vi "Update Graphs.vi"(8 "error in (no error)":errorcluster, 10 "image":variant[][](array[variant]), 11 "Detail Graph in":refnum<class "Detail Graph.lvclass">) -> (0 "error out":errorcluster, 1 "Cursor.Cursor Position":T1, 3 "Detail Graph out":refnum<class "Detail Graph.lvclass">)   [LabVIEW 2023, in "Detail Graph.lvclass"]
uses:
  Detail Graph.lvclass
  <vilib>/Utility/miscctls.llb/LVPointDoubleTypeDef.ctl
  Base Graph/Base Graph.lvclass/Base Graph.ctl
  Detail Graph.lvclass/Detail Graph.ctl
  Base Graph/Base Graph.lvclass
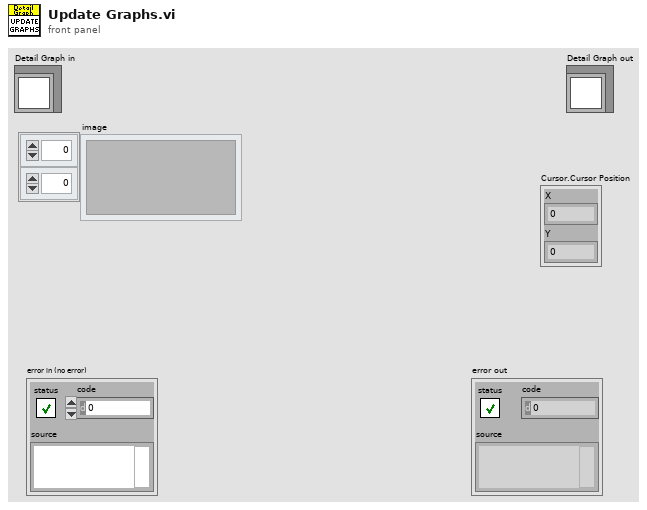
[diagram p1: front panel]
types:
  T1 = typedef "LVPointDoubleTypeDef.ctl" = cluster{"X":dbl, "Y":dbl}
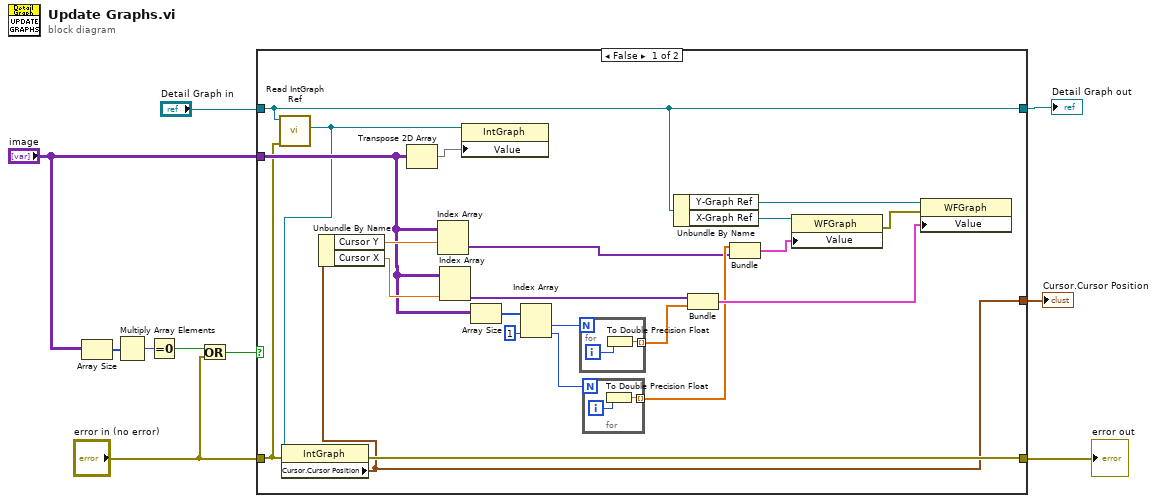
[diagram p0: block diagram]
diagram:
  n1 = Array Size(array="image") -> (size(s)=w5:i32[])
  n2 = Multiply Array Elements(1:w5) -> (0:w8:i32)
  n3 = Equal To 0?(x=w8) -> (x = 0?=w6:bool)
  n4 = Or(x=w6, y="error in (no error)") -> (x .or. y?=w7:bool)
  n5 = case shown="False" w7 {
    tunnel: [w14 w37] -> w10
    tunnel: [w22 w38] -> w2
    tunnel: "Detail Graph in" -> [w22 w38]
    tunnel: "image" -> [w23 _]
    tunnel: "error in (no error)" -> [w11 w37]
    tunnel: [w12 _] -> w1
    frame False {
      n6 = call "Read IntGraph Ref.vi"("error in (no error)"=w11, "TG Base Graph in"=w22) -> ("IntGraph Ref"=w13:refnum<vi>)  [unwired: 7 in, 2 out]
      n7 = property class="IntGraph"(reference=w13, error in=w11) -> (error out=w14:errorcluster, "Cursor.Cursor Position"=w12:T1)  [unwired: 1 out]
      n8 = Unbundle By Name(w12) -> ("Cursor Y"=w29:dbl, "Cursor X"=w26:dbl)
      n9 = Transpose 2D Array(2D array=w23) -> (transposed array=w30:variant[][])
      n10 = Index Array(array=w23, index (row)=w29) -> (element=w15:variant[])  [unwired: 1 in]
      n11 = Index Array(array=w23, index (col)=w26) -> (element=w24:variant[])  [unwired: 1 in]
      n12 = property class="IntGraph"(reference=w13, "Value"=w30) -> ()  [unwired: 1 in, 2 out]
      n13 = Array Size(array=w23) -> (size(s)=w32:i32[])
      n14 = Index Array(array=w32, index #2=1 ("index")) -> (element #1=w31:i32, element #2=w27:i32)  [unwired: 1 in]
      n15 = for {
        N: w31 -> [_]
        tunnel: [w36] -> w25 mode=indexing
        i -> [w35]
        n16 = To Double Precision Float(number=w35) -> (double precision float=w36:dbl)
      }
      n17 = for {
        N: w27 -> [_]
        tunnel: [w33] -> w16 mode=indexing
        i -> [w34]
        n18 = To Double Precision Float(number=w34) -> (double precision float=w33:dbl)
      }
      n19 = Unbundle By Name(w22) -> ("Y-Graph Ref"=w21:refnum<vi>, "X-Graph Ref"=w19:refnum<vi>)
      n20 = Bundle("image"=w24, w25) -> (w17:cluster{"image":variant[], dbl[]})  [unwired: 1 in]
      n21 = Bundle(w16, "image"=w15) -> (w18:cluster{dbl[], "image":variant[]})  [unwired: 1 in]
      n22 = property class="WFGraph"(reference=w19, "Value"=w18) -> (error out=w20:errorcluster)  [unwired: 1 in, 1 out]
      n23 = property class="WFGraph"(reference=w21, error in=w20, "Value"=w17) -> ()  [unwired: 2 out]
    }
    frame True {
    }
  }
  "error out" <- w10
  "Detail Graph out" <- w2
  "Cursor.Cursor Position" <- w1
